vi "Save Data.vi"(8 "error in (no error)":errorcluster, 11 "Data":waveform(dbl)[](array[waveform])) -> (0 "error out":errorcluster)   [LabVIEW 2014]
doc: "Saves data to disk in the TDMS file format."
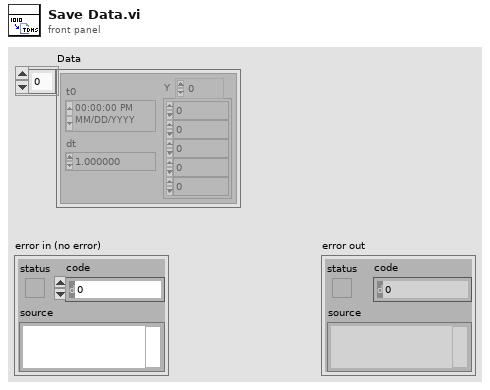
[diagram p1: front panel]
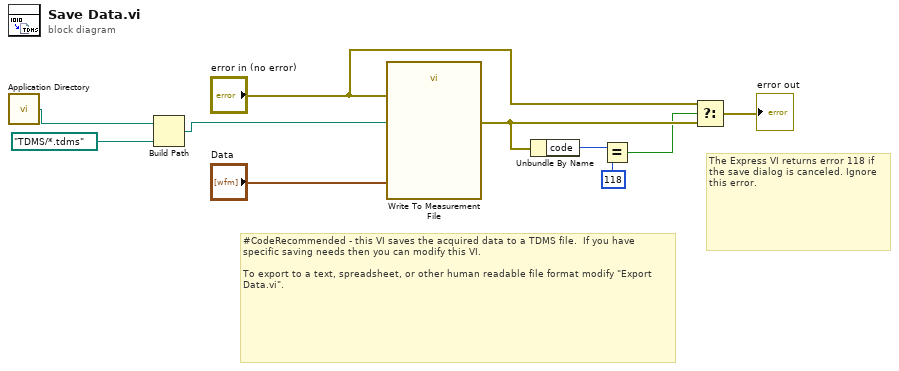
[diagram p0: block diagram]
diagram:
  # "The Express VI returns error 118 if the save dialog is canceled. Ignore this error."
  # "#CodeRecommended - this VI saves the acquired data to a TDMS file.  If you have specific saving needs then you can modify this VI.\n\nTo export to a text, spreadsheet, or other human readable file format modify \"Export Data.vi\"."
  n1 = call <vilib>:"Application Directory.vi"() -> ("Application Directory"=w2:path)
  n2 = Build Path(base path=w2, name or relative path=path "TDMS/*.tdms") -> (appended path=w1:path)
  n3 = call "Write To Measurement File"("Signals"="Data", "error in (no error)"="error in (no error)", "Filename"=w1) -> ("error out"=w8:errorcluster)  [unwired: 14 in, 2 out]
  n4 = Unbundle By Name(w8) -> ("code"=w6:i32)
  n5 = Equal?(x=w6, y=118) -> (x = y?=w5:bool)
  n6 = Select(t="error in (no error)", s=w5, f=w8) -> (s? t:f=→"error out":errorcluster)
